vi "Protocol FG.vi"(7 "Action":T1, 8 "error in (no error)":errorcluster, 10 "Protocol":string(combo), 11 "Device Item Ref in":T2 format="%.0x") -> (0 "error out":errorcluster, 2 "Protocol out":string(combo), 3 "Item Ref out":T2 format="%.0x")   [LabVIEW 2018, in "Instrument Addon Shared.lvlib"]
uses:
  Instrument Addon Shared.lvlib
  <vilib>/NI Veristand/Custom Device API/Custom Device Item Ref.ctl
  Types/FG Control.ctl
  Constants.vi
  <vilib>/NI/NI VeriStand Advanced SysDef API/_SubVIs/SysDef.Property.Get.String.vi
  <vilib>/NI/NI VeriStand Advanced SysDef API/_SubVIs/SysDef.Property.Set.String.vi
  <vilib>/NI/NI VeriStand Advanced SysDef API/SysDef API/Advanced System Definition.lvlib
  <vilib>/NI Veristand/Custom Device API/Custom Device API.lvlib
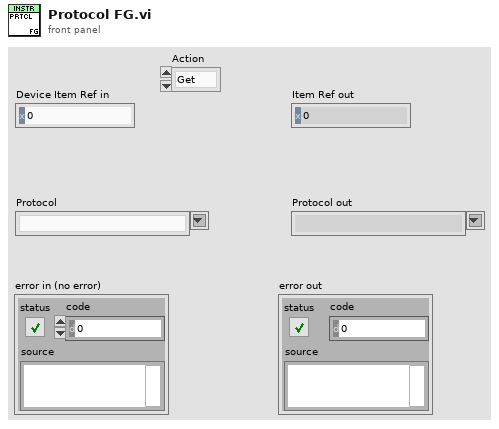
[diagram p1: front panel]
types:
  T1 = typedef "Instrument Addon Shared.lvlib/FG Control.ctl" = enum16{"Get", "Set"}
  T2 = typedef "Custom Device API.lvlib/Custom Device Item Ref.ctl" = u64
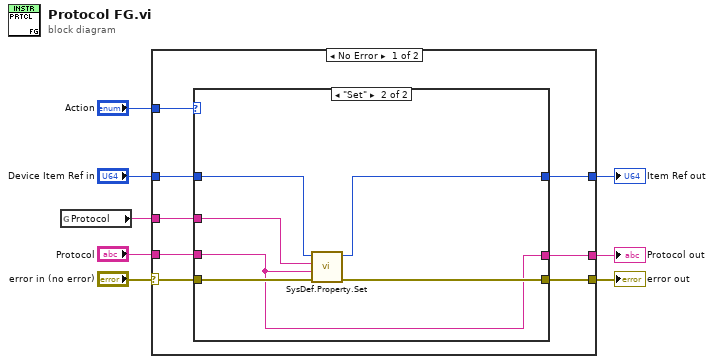
[diagram p0: block diagram]
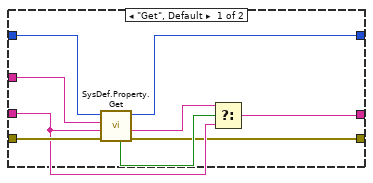
[diagram p2: hidden frame]
diagram:
  n1 = global read "Constants.vi" "Protocol"() -> (w8:string)
  n2 = case shown="No Error" "error in (no error)" {
    selector: "error in (no error)" -> [w11 w34]
    tunnel: w8 -> [w16 _]
    tunnel: [w15 w32] -> w7
    tunnel: "Device Item Ref in" -> [w14 w32]
    tunnel: "Protocol" -> [w13 w33]
    tunnel: [w12 w34] -> w4
    tunnel: [w10 w33] -> w2
    tunnel: "Action" -> [w9 _]
    frame No Error {
      n3 = case shown="\"Set\"" w9 {
        tunnel: w16 -> [w22 w31]
        tunnel: [w23 w30] -> w15
        tunnel: w14 -> [w24 w29]
        tunnel: w13 -> [w19 w26]
        tunnel: [w18 w28] -> w12
        tunnel: w11 -> [w25 w27]
        tunnel: [w17 w26] -> w10
        frame "Get", Default {
          n4 = call-poly <vilib>:"SysDef.Property.Get.vi"("error in (no error)"=w25, "Value"=w19, "Property Name"=w22, "nodeID"=w24) -> ("error out"=w18:errorcluster, "Value out"=w20:string, "nodeID out"=w23:u64, "Found?"=w21:bool)  [unwired: 4 in]
          n5 = Select(t=w20, s=w21, f=w19) -> (s? t:f=w17:string)
        }
        frame "Set" {
          n6 = call-poly <vilib>:"SysDef.Property.Set.vi"("error in (no error)"=w27, "Value"=w26, "Property Name"=w31, "nodeID"=w29) -> ("error out"=w28:errorcluster, "nodeID out"=w30:u64)  [unwired: 6 in]
        }
      }
    }
    frame Error {
    }
  }
  "Item Ref out" <- w7
  "error out" <- w4
  "Protocol out" <- w2
